vi "Start Engine.vi"(7 "Engine Type":refnum<class "LQCoreEngine.lvclass">, 8 "Error In":errorcluster, 10 "Command Line Args (\"\")":string) -> (0 "Error Out":errorcluster, 3 "New Engine":refnum<class "LQCoreEngine.lvclass">)   [LabVIEW 2014, in "LQ Core.lvlib" / "LQCoreEngine.lvclass"]
doc: "Starts the LQ engine. This VI must be called before most other LQ VIs.\n\nThe <b>Engine Type</b> input determines the number of properties that will be made available to you (where LQCoreEngine is the most basic while LQWidgetEngine is the most comprehensive).\n\nThe <b>Command Line Args</b> input provides a low-level way to fine-tune the LQ engine. For a list of supported arguments, see the documentation for the constructors of QApplication and QGuiApplication (this VI's <b>Detailed Help</b> links to the former)."
uses:
  LQCoreEngine.lvclass
  _Internal/LQIdentity Registry Action.ctl
  LQIdentity/LQIdentity.lvclass/LQIdentity.ctl
  _Private/Signals and Slots/Connection Action.ctl
  _Private/Global Quit Event Holder.vi
  LQ Core.lvlib
  LQIdentity/LQIdentity.lvclass
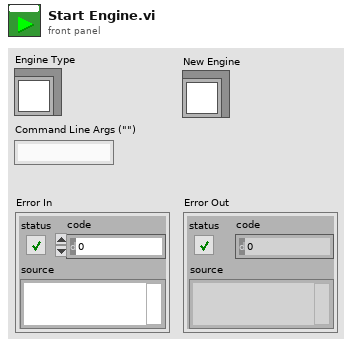
[diagram p1: front panel]
types:
  T1 = typedef "LQ Core.lvlib/LQCoreEngine.lvclass/LQIdentity Registry Action.ctl" = enum16{"Init", "Register LQIdentity", "Get LQIdentity Info", "Deregister LQIdentity"}
  T2 = typedef "LQ Core.lvlib/LQCoreEngine.lvclass/Connection Action.ctl" = enum16{"Init", "Add Connection", "Get Connections", "Clean Up"}
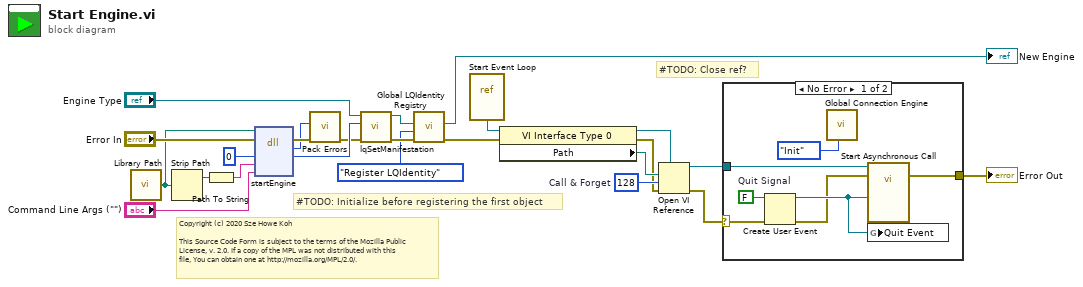
[diagram p0: block diagram]
diagram:
  w23 = 128  # Call & Forget
  # "Copyright (c) 2020 Sze Howe Koh\n\nThis Source Code Form is subject to the terms of the Mozilla Public\nLicense, v. 2.0. If a copy of the MPL was not distributed with this\nfile, You can obtain one at http://mozilla.org/MPL/2.0/."
  # "#TODO: Initialize before registering the first object"
  # "#TODO: Close ref?"
  n1 = call "Library Path.vi"() -> ("Library Path"=w18:path)
  n2 = Strip Path(path=w18) -> (stripped path=w17:path)  [unwired: 1 out]
  n3 = Path To String(path=w17) -> (string=w16:string)
  n4 = dll-call lib="?" fn="startEngine"(path in=w18, error in="Error In", "_retVal"=u64 0, "pluginDir"=w16, "cliArgs"="Command Line Args (\"\")") -> (error out=w15:errorcluster, "errorCode"=w14:i32, "_retVal"=w8:u64)  [unwired: 3 in, 1 out]
  n5 = call "Pack Errors.vi"("Error In"=w15, "Error Code"=w14) -> ("Error Out"=w7:errorcluster)  [unwired: 9 in]
  n6 = call "lqSetManifestation.vi"("Error In"=w7, "Manifestation"=w8, "LQIdentity in"="Engine Type") -> ("Error Out"=w10:errorcluster, "LQIdentity out"=w11:refnum<class "LQCoreEngine.lvclass">)  [unwired: 7 in]
  n7 = call "Global LQIdentity Registry.vi"("Error In"=w10, "Registry Action"=LQIdentity_Registry_Action."Register LQIdentity", "LQIdentity Info In"=w11) -> ("Error Out"=w2:errorcluster, "LQIdentity Info Out"=→"New Engine":refnum<class "LQCoreEngine.lvclass">)  [unwired: 7 in]
  n8 = vi-ref "Start Event Loop.vi"() -> (w20:refnum<vi>)
  n9 = property class="VI Interface Type 0"(reference=w20, error in=w2) -> (reference out=w21:refnum<vi>, error out=w19:errorcluster, "Path"=w22:path)
  n10 = Open VI Reference(type specifier VI Refnum (for type only)=w21, vi path=w22, options=w23, error in (no error)=w19) -> (vi reference=w5:refnum<vi>, error out=w13:errorcluster)  [unwired: 2 in]
  n11 = case shown="No Error" w13 {
    selector: w13 -> [w30 w32]
    tunnel: w5 -> [w29 _]
    tunnel: [w26 w32] -> w4
    frame No Error {
      w31 = FALSE  # Quit Signal
      n12 = Create User Event(user event datatype=w31, error in=w30) -> (user event=w28:refnum<user-event>, error out=w27:errorcluster)
      n13 = call "Global Connection Engine.vi"("Connection Action"=Connection_Action."Init") -> ()  [unwired: 10 in, 1 out]
      n14 = call-by-ref "Start Asynchronous Call"(reference=w29, error in=w27, "Quit Event"=w28) -> (error out=w26:errorcluster)  [unwired: 11 in, 1 out]
      n15 = global write "Global Quit Event Holder.vi" "Quit Event"(w28) -> ()
    }
    frame Error {
    }
  }
  "Error Out" <- w4
